vi "Dashboard Main.vi"() -> ()   [LabVIEW 2019]
uses:
  <vilib>/Utility/miscctls.llb/LVRowAndColumnTypeDef.ctl
  <vilib>/event_ctls.llb/eventvkey.ctl
  <vilib>/Rock Robotics/Network Tables/NT Read Numeric Array.vi
  <vilib>/Rock Robotics/Network Tables/NT Read Boolean.vi
  <vilib>/Rock Robotics/WPI/Dashboard/WPI_DashboardLogging Global.vi
panel:
  in  "Camera Settings Right":T1={"Frame Rate"=30, "Compression"=30, "Size"=1, "DB Camera Config"=FALSE} {"Frame Rate" scale=1.0..30.0; "Compression" scale=100.0..-1.0; "Size" items=["640x480", "320x240", "160x120"]}
  in  "Camera Name Right":string(combo)="No Camera Selection"
  out "Camera Perf":string
  in  "Camera Settings":T1={"Frame Rate"=30, "Compression"=30, "Size"=1, "DB Camera Config"=FALSE} {"Frame Rate" scale=1.0..30.0; "Compression" scale=100.0..-1.0; "Size" items=["640x480", "320x240", "160x120"]}
  in  "TCP":refnum<k5>
  in  "Rec Mode":enum32{"Stop", "Record", "Playback"}(radio)
  out "Robot IP":string
  out "Image Message":string="Timeout in Camera Communications"
  in  "Dashboard Tab":T2(tab)
  in  "Select Auto":string(combo)="Select Autonomous ..."
  out "NT Connection":bool
  out "MotorChart R":cluster{"Numeric":dbl, "Numeric":dbl}(graph)
  out "MotorChart L":cluster{"Numeric":dbl, "Numeric":dbl}(graph)
  out "MotorSliders R":cluster{"MotorSlide1":dbl, "MotorSlide2":dbl} {"MotorSlide2" scale=-1.0..1.0 scale format="%#_2e"; "MotorSlide1" scale=-1.0..1.0 scale format="%#_2e"}
  out "MotorSliders L":cluster{"MotorSlide1":dbl, "MotorSlide2":dbl} {"MotorSlide2" scale=-1.0..1.0 scale format="%#_2e"; "MotorSlide1" scale=-1.0..1.0 scale format="%#_2e"}
  out "Gyro":dbl(knob) scale=0.0..360.0
  out "JS1 Z":dbl(slide) scale=-1.0..1.0 scale format="%#_2e"
  out "JS1 Graph":cluster{"X":dbl, "Y":dbl}[](graph)
  out "JS1 Buttons":T3
  out "JS2 Z":dbl(slide) scale=-1.0..1.0 scale format="%#_2e"
  out "JS2 Graph":cluster{"X":dbl, "Y":dbl}[](graph)
  out "JS2 Buttons":T3
  out "Mode":T4(ring)=enum."Auto Disabled"
  out "Right Camera Perf":cluster{"Bandwidth (Mbps)":dbl, "FPS":dbl}
  out "Camera Image Right":T5(plugin-control)
  in  "DB/String 9":string
  in  "DB/String 8":string
  in  "DB/String 7":string
  in  "DB/String 6":string
  in  "DB/String 5":string
  in  "DB/String 4":string
  in  "DB/String 3":string
  in  "DB/String 2":string
  in  "DB/String 1":string
  in  "DB/String 0":string
  in  "DB/Slider 0":dbl(slide) scale=0.0..5.0
  in  "DB/Slider 1":dbl(slide) scale=0.0..5.0
  in  "DB/Slider 2":dbl(slide) scale=0.0..5.0
  in  "DB/Slider 3":dbl(slide) scale=0.0..5.0
  out "DB/LED 3":bool
  out "DB/LED 2":bool
  out "DB/LED 1":bool
  out "DB/LED 0":bool
  in  "DB/Button 3":bool
  in  "DB/Button 2":bool
  in  "DB/Button 1":bool
  in  "DB/Button 0":bool caption="New Name"
  out "Intake rotation":dbl(knob) scale=-100.0..100.0
  out "version_note":string
  in  "FIRE PULSE":dbl=0.4 caption="PULSE (s)" min=0.1 max=1.0 step=0.05 format="%#.1g"
  in  "FIRE SPD":dbl=0.4 min=0.4 max=1.0 step=0.1 format="%#.1g"
  out "GAME COLOR":u32(colorbox)
  out "SENSOR COLOR":u32(colorbox)
  out "DRIVER Z":dbl
  out "DRIVER Y":dbl
  out "SHOOTER HT":dbl[](array[slide]) caption="SHOOTER Ht & Spd" scale=0.2..1.0
  out "CW ROTATION":bool
  out "CW DEPLOY":bool
  out "LIFT LOCK":bool
  out "INV DRIVE":bool
  out "FORZA":bool
  out "1 Joystick":bool
  out "NEO MOTOR TEMPS":dbl[](array[slide]) scale=70.0..300.0
  in  "HEIGHT":i32
  in  "TOP":i32
  in  "WIDE":i32
  in  "LEFT":i32
  in  "Test Slider":dbl(slide) scale=0.0..100.0 scale format="%#_3g"
  in  "On/Off":bool caption="Solenoid"
  in  "Test Name":u16(ring) items=["Select the test to run..."]
  in  "Test Tree":string(tree)
  in  "Motor":cluster{"Value":dbl, "Enable":bool} {"Value" scale=-1.0..1.0 scale format="%#_3g"}
  out "Progress":T6 {"Test Progress" scale=0.0..100.0}
  in  "Rev/Fwd":cluster{"Forward":bool, "Reverse":bool}
  in  "Test Ring":u16(ring) items=["Monochrome", "Color"]
  out "Cmd Status":string
  in  "Execute Command":bool
  in  "Command Params":string[][](table)
  in  "Command Selection":i32(listbox)
  in  "CheckList":i32(listbox)
  out "Tree":string(tree)
  out "Camera Image":T5(plugin-control)
  out "Background":bool
  in  "Camera Name":string(combo)="No Camera Selection"
  # "HW"
  # "HW"
  # "Joysticks"
  # "Drive Motors"
  # "Front"
  # "Right"
  # "Left"
  # "Back"
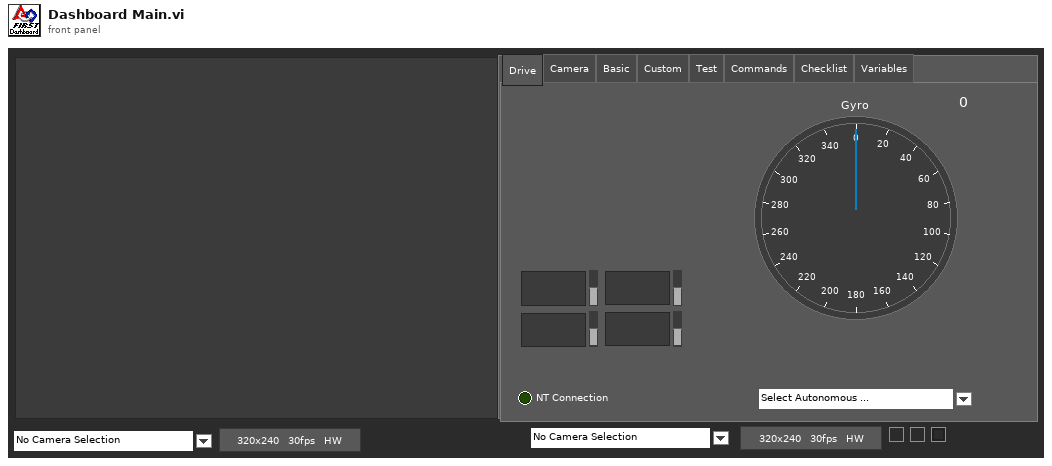
[diagram p1: front panel]
types:
  T1 = cluster{"Frame Rate":i32, "Compression":i32, "Size":u16, "DB Camera Config":bool}
  T2 = enum32{"Drive", "Camera", "Basic", "Custom", "Test", "Commands", "Checklist", "Variables"}
  T3 = cluster{bool, bool, bool, bool, bool, bool, bool, bool, bool, bool, bool, bool}
  T4 = enum8{"Tele-Op Disabled", "Tele-Op Enabled", "Auto Disabled", "Auto Enabled", "Test Disabled", "Test Enabled", "Disconnected", "No Code", "E-Stop"}
  T5 = typedef "IMAQ Image.ctl" = refnum<image>
  T6 = cluster{"Test Progress":u8, "Test Progress Text":string}
  T7 = cluster{"Save Path":path, "Interval (s)":dbl, "Keep":i32}
  T8 = typedef "Image Type" = u32
  T9 = cluster{"IDs":cluster{"RPC field ID":u16, "Unique ID":u16}, "String":string}
  T10 = cluster{"Error Strings":string, "Disable Counts":cluster{u16, u16}, "Rail Faults":cluster{u16, u16, u16}, "Robot IP":string, "DB Mode":u8, "Event Info":cluster{"Name":string, "Type":u8, "Number":u16, "Replay":u8}}
  T11 = cluster{"Storage":cluster{"Disk Free":u64, "RAM Block":u32, "RAM free":u32}, "CPU Utilization":cluster{"CPU % ISR":sgl, "CPU % Time Crit":sgl, "CPU % Timed Str":sgl, "CPU % High":sgl, "CPU % Above":sgl, "CPU % Normal":sgl, "CPU % Low":sgl}, "CAN":cluster{"% Bus Utilization":sgl, "Bus Off Cnt":u32, "TX_FIFO Full Cnt":u32, "Receive Error Cnt":u8, "Transmit Error Cnt":u8}, "HID":cluster{"HID Outputs":u32, "Rumble Low":u16, "Rumble High":u16}[]}
  T12 = cluster{"Status bits":cluster{"Test Mode":bool, "Autonomous":bool, "Enabled":bool, "Code Start":bool, "Brownout":bool, "Reserved 2":bool, "Reserved 3":bool, "E-Stop":bool}, "Code Trace":cluster{"Disabled":bool, "TeleOp":bool, "Auto":bool, "Test":bool}, "Controller Type":enum16{"unknown", "cRIO", "roboRio"}, "Code?":enum16{"unknown", "noCode", "code"}, "Battery V":dbl}
  T13 = cluster{"Control Bits":cluster{"TestMode":bool, "Autonomous":bool, "Enabled":bool, "FMS Present":bool, bool, bool, bool, "E-Stop":bool}, "Team Station ":u8, "Countdown":sgl, "Joystick Values":cluster{"Axes":dbl[], "Buttons":bool[], "POVs":i16[]}[]}
  T14 = cluster{"Axes":dbl[], "Buttons":bool[], "POVs":i16[]}[]
  T15 = cluster{"Axes":dbl[], "Buttons":bool[], "POVs":i16[]}
  T16 = cluster{"Buttons[0]":bool, "Buttons[1]":bool, "Buttons[2]":bool, "Buttons[3]":bool, "Buttons[4]":bool, "Buttons[5]":bool, "Buttons[6]":bool, "Buttons[7]":bool, "Buttons[8]":bool, "Buttons[9]":bool, "Buttons[10]":bool, "Buttons[11]":bool}
  T17 = cluster{"Camera Image":refnum<vi>, "Dashboard Tab":refnum<vi>, "Background":refnum<vi>, "Rec Mode":refnum<vi>, "Test Slider":refnum<vi>, "On/Off ":refnum<vi>, "Test Ring":refnum<vi>, "Rev/Fwd":refnum<vi>, "Test Name":refnum<vi>, "Motor":refnum<vi>, "Progress":refnum<vi>, "CheckList":refnum<vi>, "Tree":refnum<vi>, "Test Tree":refnum<vi>, "Command Params":refnum<vi>, "Command Selection":refnum<vi>, "Execute Command":refnum<vi>, "Cmd Status":refnum<vi>, "Camera Settings":refnum<vi>, "Camera Name":refnum<vi>, "Camera Perf":refnum<vi>, "Camera Settings Right":refnum<vi>, "Camera Name Right":refnum<vi>, "Camera Image Right":refnum<vi>}
  T18 = cluster{"Global Rectangle":i32[], "Contours":cluster{"Contour Type":u32, "ROI Type":u32, "Points":i32[]}[]}
  T19 = cluster{"Left":i32, "Top":i32, "Right":i32, "Bottom":i32}
  T20 = cluster{"Camera Name":string, string, "Saved DB Images Info":cluster{"Save Path":path, "Interval (s)":dbl, "Keep":i32}}
  T21 = cluster{"Camera Name Right":string, string, "Saved DB Images Info":cluster{"Save Path":path, "Interval (s)":dbl, "Keep":i32}}
  T22 = cluster{"Operation":enum16{"Update", "Clear"}, "Color Box":u32}[]
  T23 = typedef "eventvkey.ctl" = enum16{"ASCII", "Enter", "Return", "Shift", "Ctrl", "Alt", "Cmd", "Opt", "Caps", "NumLock", "Clear", "Break", "Up", "Down", "Left", "Right", "Insert", "Delete", "Home", "End", "PageUp", "PageDown", "Escape", "Help", "Pause", "ScrollLock", "F1", "F2", "F3", "F4", "F5", "F6", "F7", "F8", "F9", "F10", "F11", "F12", "F13", "F14", "F15", "F16", "F17", "F18", "F19", "F20", "F21", "F22", "F23", "F24", "Play", "VolumeUp", "VolumeDown", "Mute", "Two Byte Char"}
  T24 = cluster{"Image Size":bool, "Image Type":bool, "Pixel Value":bool, "ROI Information":bool, "Zoom Factor":bool}
  T25 = cluster{"Operation":enum16{"Update", "Clear"}, "Color Box":u32}
  T26 = typedef "LVRowAndColumnTypeDef.ctl" = cluster{"Row":i32, "Column":i32}
  T27 = cluster{"Shift":bool, "Ctrl":bool, "Alt":bool, "Cmd":bool, "Opt":bool}
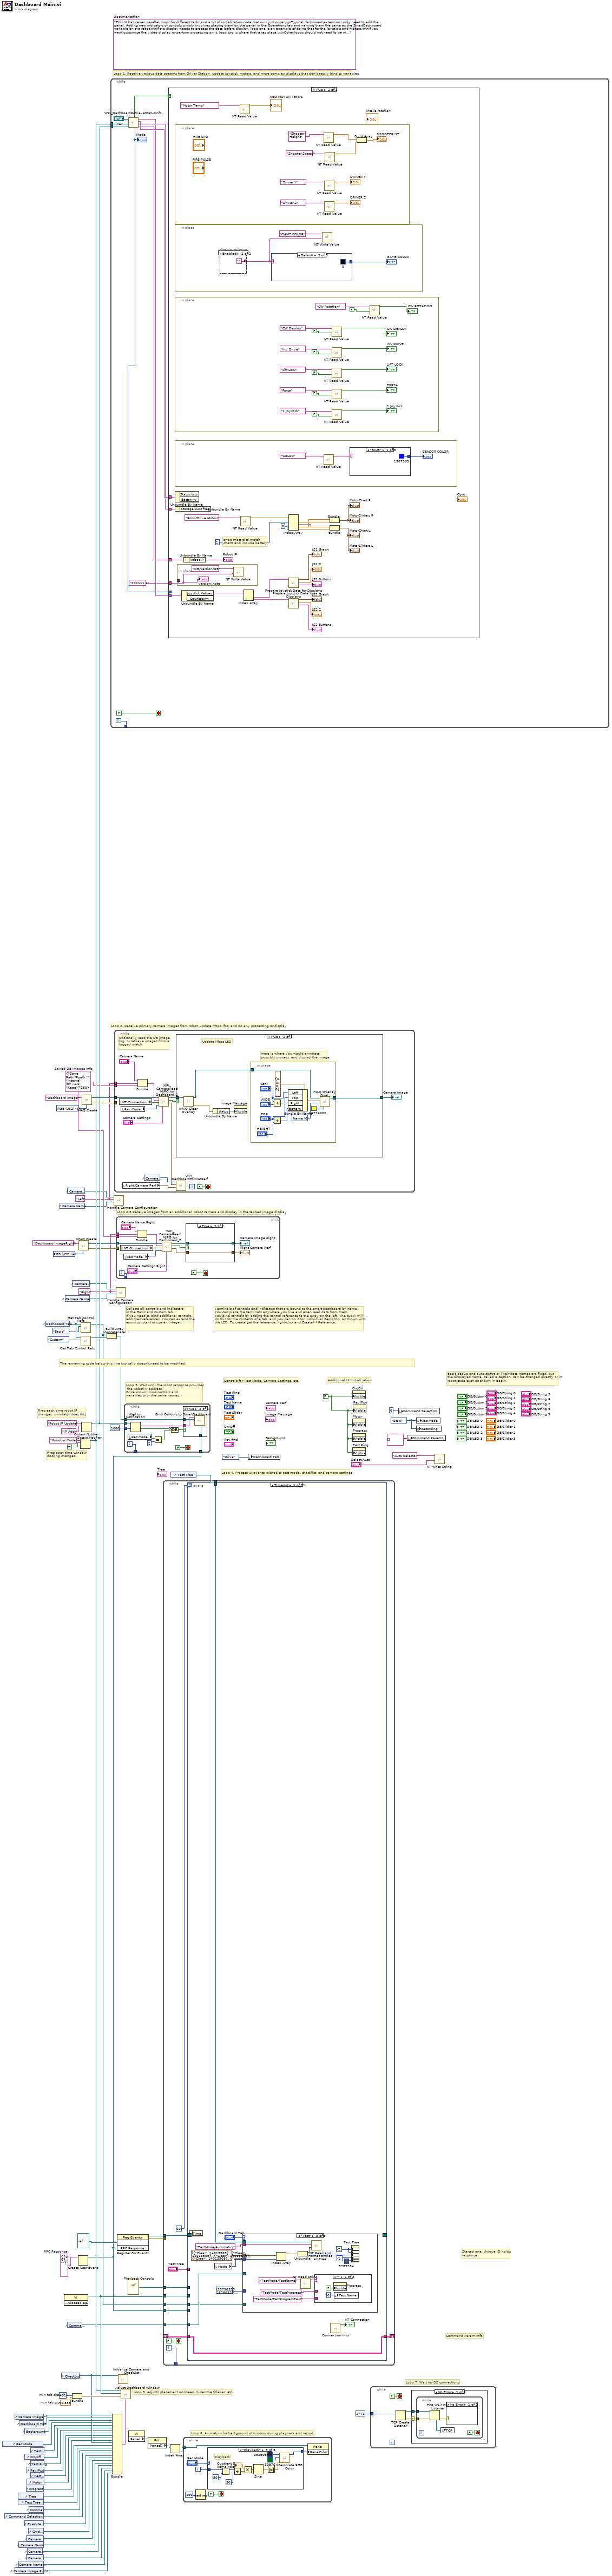
[diagram p0: block diagram]
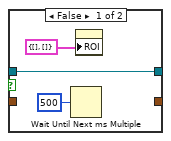
[diagram p2: hidden frame]
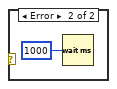
[diagram p3: hidden frame]
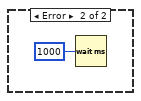
[diagram p4: hidden frame]
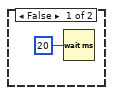
[diagram p5: hidden frame]
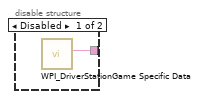
[diagram p6: hidden frame]
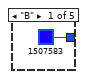
[diagram p7: hidden frame]
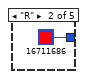
[diagram p8: hidden frame]
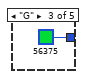
[diagram p9: hidden frame]
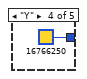
[diagram p10: hidden frame]
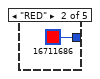
[diagram p11: hidden frame]
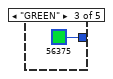
[diagram p12: hidden frame]
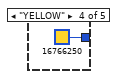
[diagram p13: hidden frame]
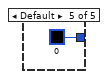
[diagram p14: hidden frame]
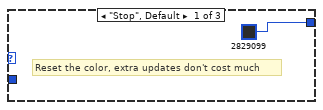
[diagram p15: hidden frame]
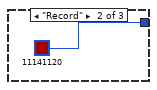
[diagram p16: hidden frame]
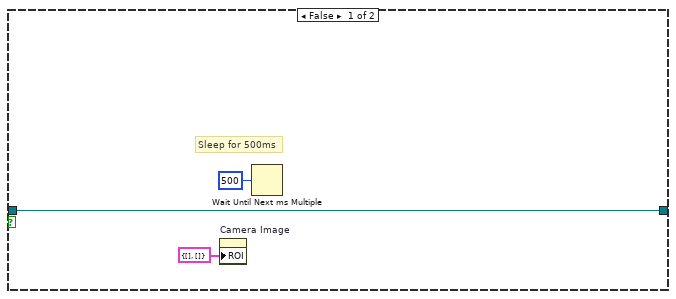
[diagram p18: hidden frame]
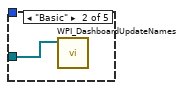
[diagram p20: hidden frame]
diagram:
  w3 = T7 {"Save Path"=path "", "Interval (s)"=1.0, "Keep"=180}  # Saved DB Images Info
  w2 = "Right"
  w1 = "Left"
  w13 = T8 4 items=["Grayscale (U8)", "Grayscale (I16)", "Grayscale (SGL)", "Complex (CSG)", "RGB (U32)", "HSL (U32)", "RGB (U64)"] ("Image Type")
  w29 = T9 {"IDs"={"RPC field ID"=0, "Unique ID"=0}, "String"=""}  # RPC Response
  w52 = 491  # min tab size
  w51 = 1.333  # min tab size
  w59 = enum32{"Stop", "Record", "Playback"}."Stop" ("Rec Mode")
  w36 = FALSE ("Visible")
  (unwired) "This VI has seven parallel loops for different tasks and a bit of initialization code that runs just once.\n\nTypical dashboard extensions only need to edit the panel. Adding new indicators or controls simply involves placing them on the panel in the Operations tab and naming them the same as the SmartDashboard variable on the robot\n\nIf the display needs to process the data before display, loop one is an example of doing that for the joysticks and motors.\n\nIf you want customize the video display or perform processing on it, loop two is where that takes place.\n\nOther loops should not need to be modified. They are pretty standard, and document the task they perform."  # Documentation
  w76 = T8 4 items=["Grayscale (U8)", "Grayscale (I16)", "Grayscale (SGL)", "Complex (CSG)", "RGB (U32)", "HSL (U32)", "RGB (U64)"] ("Image Type")
  # "Loop 2.5 Receive images from an additional  robot camera and display in the tabbed image display"
  # "Command Param Info"
  # "Started one, Unique ID holds\nresponse"
  # "Loop 7. Wait for DS connections"
  # "Basic debug and auto controls: Their data names are fixed, but\nthe displayed name, called a caption, can be changed directly or in\nrobot code such as shown in Begin."
  # "Controls for Test Mode, Camera Settings, etc."
  # "Additional UI Initialization"
  # "Loop 6. Animation for background of window during playback and record"
  # "Fires each time robot IP\nchanges, simulator does this"
  # "Fires each time window\ndocking changes."
  # "Collects all controls and indicators\nin the Basic and Custom tab.\nIf you need to bind additional controls,\nadd their references. You can extend the\nenum constant or use an integer."
  # "The remaining code below this line typically doesn't need to be modified."
  # "Loop 4. Process UI events related to test mode, checklist, and camera settings"
  # "Terminals of controls and indicators that are bound to the smart dashboard by name.\nYou can place the terminals anywhere you like and even read data from them.\nYou bind controls by adding the control reference to the array on the left. The subVI will\ndo this for the contents of a tab, and you can do it for individual items too, as shown with\nthe LED. To create get the reference, right-click and Create>>Reference."
  # "Loop 3. Wait until the robot response provides\n the Robot IP address.\nOnce known, bind controls and\nvariables with the same names."
  # "Loop 5. Adjusts placement onscreen, hides the titlebar, etc."
  # "Loop 1. Receive various data streams from Driver Station, update joystick, motors, and more complex displays that don't easily bind to variables."
  # "Loop 2. Receive primary camera images from robot, update Mbps, fps, and do any processing or display"
  n1 = control-ref of="Rec Mode"() -> (w42:refnum<vi>)
  n2 = control-ref of="Command Selection"() -> (w28:refnum<vi>)
  n3 = control-ref of="Camera Image Right"() -> (w6:refnum<vi>)
  n4 = control-ref of="Camera Image"() -> (w54:refnum<vi>)
  n5 = control-ref of="Tree"() -> (w46:refnum<vi>)
  n6 = control-ref of="Test Tree"() -> (w45:refnum<vi>)
  n7 = control-ref of="Camera Name"() -> (w19:refnum<vi>)
  n8 = control-ref of="Camera Name Right"() -> (w7:refnum<vi>)
  n9 = control-ref of="Dashboard Tab"() -> (w53:refnum<vi>)
  n10 = control-ref of="Execute Command"() -> (w30:refnum<vi>)
  n11 = control-ref of="Background"() -> (w49:refnum<vi>)
  n12 = control-ref of="On/Off"() -> (w40:refnum<vi>)
  n13 = control-ref of="Progress"() -> (w37:refnum<vi>)
  n14 = control-ref of="Camera Settings"() -> (w20:refnum<vi>)
  n15 = control-ref of="Camera Settings Right"() -> (w8:refnum<vi>)
  n16 = control-ref of="Rev/Fwd"() -> (w38:refnum<vi>)
  n17 = control-ref of="Motor"() -> (w43:refnum<vi>)
  n18 = control-ref of="Camera Perf"() -> (w18:refnum<vi>)
  n19 = control-ref of="Cmd Status"() -> (w24:refnum<vi>)
  n20 = control-ref of="Command Params"() -> (w31:refnum<vi>)
  n21 = control-ref of="Test Slider"() -> (w41:refnum<vi>)
  n22 = control-ref of="Test Ring"() -> (w39:refnum<vi>)
  n23 = control-ref of="Test Name"() -> (w44:refnum<vi>)
  n24 = control-ref of="Dashboard Tab"() -> (w57:refnum<vi>)
  n25 = control-ref of="Camera Name"() -> (w21:refnum<vi>)
  n26 = control-ref of="CheckList"() -> (w47:refnum<vi>)
  n27 = property class="VI" props=["Front Panel.Closeable"]() -> (reference out=w58:refnum<vi>)  [unwired: 2 in, 2 out]
  n28 = control-ref of="Camera Name Right"() -> (w9:refnum<vi>)
  n29 = control-ref of="Camera Settings"() -> (w22:refnum<vi>)
  n30 = control-ref of="Command Params"() -> (w23:refnum<vi>)
  n31 = control-ref of="Camera Settings Right"() -> (w10:refnum<vi>)
  n32 = Bundle("min tab size"=w52, "min tab size"=w51) -> (w50:cluster{"min tab size":i32, "min tab size":dbl})  [unwired: 1 in]
  n33 = Create User Event(user event datatype=w29) -> (user event=w25:refnum<user-event>)  [unwired: 1 in, 1 out]
  n34 = call "IMAQ Create"("Image Name"="Dashboard ImageRight", "Image Type"=w13) -> ("New Image"=w12:T5, "error out"=w11:errorcluster)  [unwired: 2 in, 1 out]
  n35 = Obtain Notifier(name (unnamed)="Window Mode", notification data type=TRUE) -> (notifier out=w34:refnum<notifier>)  [unwired: 2 in, 2 out]
  n36 = call <vilib>:"Get Tab Control Refs.vi"("Page Index"=T2."Basic" ("Dashboard Tab"), "TabControl in"=w57) -> ("ControlsOnPage"=w17:refnum<vi>[])  [unwired: 9 in]
  n37 = call <vilib>:"Get Tab Control Refs.vi"("Page Index"=T2."Custom" ("Dashboard Tab"), "TabControl in"=w57) -> ("ControlsOnPage"=w56:refnum<vi>[])  [unwired: 9 in]
  n38 = Obtain Notifier(name (unnamed)="Robot IP Update", notification data type="IP Addr" ("name (unnamed)")) -> (notifier out=w35:refnum<notifier>)  [unwired: 2 in, 2 out]
  n39 = call "IMAQ Create"("Image Name"="Dashboard Image", "Image Type"=w76) -> ("New Image"=w74:T5, "error out"=w73:errorcluster)  [unwired: 2 in, 1 out]
  n40 = Build Array (concatenate)(w17, w56) -> (w55:refnum<vi>[])
  n41 = while {
    tunnel: [w87] -> _
    tunnel: w35 -> [w81]
    tunnel: w34 -> [w78]
    i -> [w87]
    stop <- FALSE stop-if-true
    n42 = call <vilib>:"WPI_DashboardRetrieveStatusInfo.vi"("Binding Refnum"=w81, "Window Mode Notifier"=w78, "TCP Cnx"="TCP") -> ("Power and Errors"=w82:T10, "Robot Metrics"=w85:T11, "Status Info"=w86:T12, "Control Info"=w83:T13, "Robot Mode"=w80:T4, "Process?"=w84:bool)  [unwired: 3 in]
    "Mode" <- w80
    n43 = case shown="True" w84 {
      tunnel: w86 -> [_ w116]
      tunnel: w85 -> [_ w115]
      tunnel: w83 -> [_ w114]
      tunnel: w82 -> [_ w113]
      tunnel: w80 -> [_ _]
      tunnel: "2021v1.2" ("version_note") -> [_ w92]
      frame False {
        n44 = Wait (ms)(milliseconds to wait=u32 20) -> ()  [unwired: 1 out]
      }
      frame True {
        # "swap motors to match\ncharts and include battery"
        n45 = in-place {
          n46 = call-poly <vilib>:"NT Read Value.vi"("Name"="Shooter Height") -> ("Numeric"=w140:dbl)  [unwired: 9 in, 1 out]
          n47 = call-poly <vilib>:"NT Read Value.vi"("Name"="Driver Y") -> ("Numeric"=→"DRIVER Y":dbl)  [unwired: 9 in, 1 out]
          n48 = call-poly <vilib>:"NT Read Value.vi"("Name"="Driver Z") -> ("Numeric"=→"DRIVER Z":dbl)  [unwired: 9 in, 1 out]
          n49 = call-poly <vilib>:"NT Read Value.vi"("Name"="Shooter Speed") -> ("Numeric"=w138:dbl)  [unwired: 9 in, 1 out]
          n50 = Build Array(w140, w138) -> (→"SHOOTER HT":dbl[])
        }
        n51 = in-place {
          n52 = disable-structure shown="Enabled" {
            disable-tunnel: [w122 "" ("Game Specific Data")] -> w119
            frame Disabled {
              n53 = call <vilib>:"WPI_DriverStationGame Specific Data.vi"() -> ("Game Specific Data"=w122:string)  [unwired: 11 in]
            }
            frame Enabled {
            }
          }
          n54 = case shown="Default" w119 {
            tunnel: [u32 1507583 ("SENSOR COLOR") u32 16711686 ("SENSOR COLOR") u32 56375 ("SENSOR COLOR") u32 16766250 ("SENSOR COLOR") u32 0 ("SENSOR COLOR")] -> w121
            frame "B" {
            }
            frame "R" {
            }
            frame "G" {
            }
            frame "Y" {
            }
            frame Default {
            }
          }
          "GAME COLOR" <- w121
          n55 = call-poly <vilib>:"NT Write Value.vi"("String"=w119, "Name"="GAME COLOR") -> ()  [unwired: 9 in, 1 out]
        }
        n56 = in-place {
          n57 = call-poly <vilib>:"NT Read Value.vi"("Default Value"=FALSE, "Name"="CW Deploy") -> ("Boolean"=→"CW DEPLOY":bool)  [unwired: 8 in, 1 out]
          n58 = call-poly <vilib>:"NT Read Value.vi"("Default Value"=FALSE, "Name"="Inv Drive") -> ("Boolean"=→"INV DRIVE":bool)  [unwired: 8 in, 1 out]
          n59 = call-poly <vilib>:"NT Read Value.vi"("Default Value"=FALSE, "Name"="Lift Lock") -> ("Boolean"=→"LIFT LOCK":bool)  [unwired: 8 in, 1 out]
          n60 = call-poly <vilib>:"NT Read Value.vi"("Default Value"=FALSE, "Name"="Forza") -> ("Boolean"=→"FORZA":bool)  [unwired: 8 in, 1 out]
          n61 = call-poly <vilib>:"NT Read Value.vi"("Default Value"=FALSE, "Name"="1 Joystick") -> ("Boolean"=→"1 Joystick":bool)  [unwired: 8 in, 1 out]
          n62 = call-poly <vilib>:"NT Read Value.vi"("Default Value"=FALSE, "Name"="CW Rotation") -> ("Boolean"=→"CW ROTATION":bool)  [unwired: 8 in, 1 out]
        }
        n63 = in-place {
          n64 = call-poly <vilib>:"NT Read Value.vi"("Name"="COLOR") -> ("String"=w130:string)  [unwired: 9 in, 1 out]
          n65 = case shown="\"BLUE\"" w130 {
            tunnel: [u32 1507583 ("SENSOR COLOR") u32 16711686 ("SENSOR COLOR") u32 56375 ("SENSOR COLOR") u32 16766250 ("SENSOR COLOR") u32 0 ("SENSOR COLOR")] -> w129
            frame "BLUE" {
            }
            frame "RED" {
            }
            frame "GREEN" {
            }
            frame "YELLOW" {
            }
            frame Default {
            }
          }
          "SENSOR COLOR" <- w129
        }
        n66 = Unbundle By Name(w116) -> ()  [unwired: 2 out]
        n67 = Unbundle By Name(w115) -> ()  [unwired: 1 out]
        n68 = in-place {
          in-place-border: w92 -> [w117]
          n69 = call-poly <vilib>:"NT Write Value.vi"("String"=w117, "Name"="DB/version/DB") -> ()  [unwired: 9 in, 1 out]
          "version_note" <- w117
        }
        n70 = Unbundle By Name(w114) -> ("Joystick Values"=w104:T14)  [unwired: 1 out]
        n71 = Unbundle By Name(w113) -> ("Robot IP"=→"Robot IP":string)
        n72 = call-poly <vilib>:"NT Read Value.vi"("Name"="Motor Temp") -> ("Numeric Array"=→"NEO MOTOR TEMPS":dbl[])  [unwired: 9 in, 1 out]
        n73 = call-poly <vilib>:"NT Read Value.vi"("Name"="RobotDrive Motors") -> ("Numeric Array"=w94:dbl[])  [unwired: 9 in, 1 out]
        n74 = Index Array(array=w104) -> (element #1=w103:T15, element #2=w99:T15)  [unwired: 2 in]
        n75 = Index Array(array=w94, index #1=1, index #4=0) -> (element #1=w108:dbl, element #2=w109:dbl, element #3=w107:dbl, element #4=w112:dbl)  [unwired: 2 in]
        n76 = call "Prepare Joystick Data for Displays.vi"("Joystick Values"=w103) -> ("Buttons"=→"JS1 Buttons":T16, "Z Axis"=→"JS1 Z":dbl, "Cartesian Data"=→"JS1 Graph":cluster{"X axis":dbl, "X axis":dbl}[])  [unwired: 8 in]
        n77 = call "Prepare Joystick Data for Displays.vi"("Joystick Values"=w99) -> ("Buttons"=→"JS2 Buttons":T16, "Z Axis"=→"JS2 Z":dbl, "Cartesian Data"=→"JS2 Graph":cluster{"X axis":dbl, "X axis":dbl}[])  [unwired: 8 in]
        n78 = Bundle("Numeric"=w107, "Numeric"=w108) -> (→"MotorChart R" →"MotorSliders R":cluster{"Numeric":dbl, "Numeric":dbl})  [unwired: 1 in]
        n79 = Bundle("Numeric"=w109, "Numeric"=w112) -> (→"MotorChart L" →"MotorSliders L":cluster{"Numeric":dbl, "Numeric":dbl})  [unwired: 1 in]
      }
    }
  }
  n80 = Bundle("Camera Image"=w54, "Dashboard Tab"=w53, "Background"=w49, "Rec Mode"=w42, "Test Slider"=w41, "On/Off"=w40, "Test Ring"=w39, "Rev/Fwd"=w38, "Test Name"=w44, "Motor"=w43, "Progress"=w37, "CheckList"=w47, "Tree"=w46, "Test Tree"=w45, "Command Params"=w31, "Command Selection"=w28, "Execute Command"=w30, "Cmd Status"=w24, "Camera Settings"=w20, "Camera Name"=w19, "Camera Perf"=w18, "Camera Settings Right"=w8, "Camera Name Right"=w7, "Camera Image Right"=w6) -> (w48:T17)  [unwired: 1 in]
  n81 = call "Handle Camera Configuration.vi"("CameraNameRef"=w21, "Display Name"=w1, "ClusterRef"=w22) -> ()  [unwired: 9 in]
  n82 = while {
    tunnel: w74 -> [w177]
    tunnel: w73 -> [_]
    tunnel: w3 -> [w170]
    tunnel: w1 -> [w167]
    stop <- FALSE stop-if-true
    # "Optionally read the DB image,\nlog, or retrieve images from a\nlogged match"
    n83 = local read "NT Connection"() -> (w171:bool)
    n84 = local read "Rec Mode"() -> (w174:enum32{"Stop", "Record", "Playback"})
    n85 = local read "Right Camera Perf"() -> (w165:cluster{"Bandwidth (Mbps)":dbl, "FPS":dbl})
    n86 = Bundle("Camera Name"="Camera Name", w167, "Saved DB Images Info"=w170) -> (w169:T20)  [unwired: 1 in]
    n87 = control-ref of="Camera Perf"() -> (w164:refnum<vi>)
    n88 = call <vilib>:"WPI_CameraRead MJPG for Dashboard_2.vi"("Camera Settings"="Camera Settings", "Rec Mode"=w174, "NT Connection"=w171, "Capture Info"=w169, "Image in"=w177) -> ("perf info"=w166:cluster{"Bandwidth (Mbps)":dbl, "fps":dbl}, "Active"=w175:bool, "Image\\ out"=w176:T5)  [unwired: 4 in]
    n89 = case shown="True" w175 {
      tunnel: w176 -> [w180 w184]
      tunnel: [w180 w182] -> w172
      frame False {
        # "Sleep for 500ms"
        n90 = property on="Camera Image" class="ImageControl"("ROI"=T18 {"Global Rectangle"=[], "Contours"=[]}) -> ()  [unwired: 2 in, 2 out]
        n91 = Wait Until Next ms Multiple(millisecond multiple=u32 500) -> ()  [unwired: 1 out]
      }
      frame True {
        # "Here is where you would annotate,\npossibly process, and display the image"
        # "Update Mbps LED"
        n92 = call "IMAQ Clear Overlay"("Image"=w184) -> ("error out"=w185:errorcluster, "Image Out"=w183:T5)  [unwired: 2 in, 7 out]
        n93 = Unbundle By Name(w185) -> ("status"=w186:bool)
        n94 = property on="Image Message" class="Str"("Visible"=w186) -> ()  [unwired: 2 in, 2 out]
        n95 = in-place {
          in-place-border: w183 -> [w198]
          in-place-border: [w197] -> w182
          w196 = u32 0 items=["Frame", "Fill"] ("Drawing Mode (Frame)")
          n96 = Add(x="LEFT", y="WIDE") -> (x+y=w193:i32)
          n97 = Add(x="TOP", y="HEIGHT") -> (x+y=w192:i32)
          n98 = Bundle By Name(cluster=T19 {"Left"=0, "Top"=0, "Right"=0, "Bottom"=0} ("Bounding Rectangle"), "Left"="LEFT", "Top"="TOP", "Right"=w193, "Bottom"=w192) -> (w194:T19)
          n99 = call "IMAQ Overlay Oval"("Color"=u32 16776002, "Drawing Mode (Frame)"=w196, "Bounding Rectangle"=w194, "Image"=w198) -> ("Image Out"=w197:T5)  [unwired: 6 in, 1 out]
        }
      }
    }
    "Camera Image" <- w172
    n100 = call <vilib>:"WPI_DashboardFormatPerf.vi"("Right Camera Perf"=w165, "Performance"=w166, "String in"=w164) -> ()  [unwired: 9 in]
  }
  n101 = call "Handle Camera Configuration.vi"("CameraNameRef"=w9, "Display Name"=w2, "ClusterRef"=w10) -> ()  [unwired: 9 in]
  n102 = while {
    tunnel: w12 -> [w213]
    tunnel: w11 -> [_]
    tunnel: [w208] -> _
    tunnel: w3 -> [w204]
    tunnel: w2 -> [w201]
    i -> [w208]
    stop <- FALSE stop-if-true
    n103 = local read "NT Connection"() -> (w205:bool)
    n104 = local read "Rec Mode"() -> (w212:enum32{"Stop", "Record", "Playback"})
    n105 = Bundle("Camera Name Right"="Camera Name Right", w201, "Saved DB Images Info"=w204) -> (w203:T21)  [unwired: 1 in]
    n106 = call <vilib>:"WPI_CameraRead MJPG for Dashboard_2.vi"("Camera Settings"="Camera Settings Right", "Rec Mode"=w212, "NT Connection"=w205, "Capture Info"=w203, "Image in"=w213) -> ("perf info"=w199:cluster{"Bandwidth (Mbps)":dbl, "fps":dbl}, "Active"=w207:bool, "Image\\ out"=w210:T5)  [unwired: 4 in]
    n107 = case shown="True" w207 {
      tunnel: w210 -> [w215 w218]
      tunnel: [w215 w218] -> w206
      tunnel: [_ w217] -> w200
      tunnel: w199 -> [_ w217]
      frame False {
        n108 = Wait Until Next ms Multiple(millisecond multiple=u32 500) -> ()  [unwired: 1 out]
        n109 = property on="Camera Image Right" class="ImageControl"("ROI"=T18 {"Global Rectangle"=[], "Contours"=[]}) -> ()  [unwired: 2 in, 2 out]
      }
      frame True {
      }
    }
    "Camera Image Right" <- w206
    "Right Camera Perf" <- w200
  }
  n110 = register-events(refnum<vi> refnum, w25) -> (reference out=w63:refnum<event-registration>, error out=w62:errorcluster)  [unwired: 2 in]
  n111 = call "Initialize Camera and CheckList.vi"("ListBox in"=w47) -> ()  [unwired: 11 in]
  n112 = call "Adjust Dashboard Window.vi"("Sizing Refnums"=w48, "Size Constraints"=w50, "VI"=w58, "WIn Mode"=w34) -> ()  [unwired: 8 in]
  n113 = while {
    tunnel: w55 -> [w230]
    tunnel: w35 -> [w228]
    tunnel: [w226] -> _
    tunnel: u32 1000 ("milliseconds to wait") -> [w225]
    tunnel: w25 -> [w219]
    i -> [w226]
    stop <- FALSE stop-if-true
    n114 = local read "Rec Mode"() -> (w221:enum32{"Stop", "Record", "Playback"})
    n115 = Wait on Notification(notifier=w228, timeout in ms (-1)=w225) -> (notification=w227:string, timed out?=w223:bool)  [unwired: 2 in, 2 out]
    n116 = Equal?(x=w221, y=u16 2 ("Rec Mode")) -> (x = y?=w222:bool)
    n117 = Compound Arithmetic op=OR(invert w223, w222) -> (w224:bool)
    n118 = case shown="True" w224 {
      tunnel: w230 -> [_ w233]
      tunnel: w227 -> [_ w232]
      tunnel: w219 -> [_ w231]
      frame False {
      }
      frame True {
        n119 = call <vilib>:"Bind Controls to SmartDashboard.vi"("RPC ref"=w231, "Bound Control Refs"=w233, "Server IP Address"=w232) -> ()  [unwired: 9 in]
      }
    }
  }
  n120 = vi-ref "Playback Controls.vi"() -> (w64:refnum<vi>)
  n121 = property class="VI"() -> ("Panel"=w66:refnum<vi>)  [unwired: 2 in, 2 out]
  n122 = property class="Pnl"(reference=w66) -> ("Panes[]"=w67:refnum<vi>[])  [unwired: 1 in, 2 out]
  n123 = Index Array(array=w67) -> (element=w65:refnum<vi>)  [unwired: 1 in]
  n124 = control-ref of="Test Tree"() -> (w68:refnum<vi>)
  n125 = while {
    tunnel: [w243] -> _
    tunnel: w68 -> [w242]
    tunnel: w64 -> [w241]
    tunnel: w63 -> [w240]
    tunnel: w62 -> [_]
    tunnel: w58 -> [w239]
    tunnel: w25 -> [w238]
    tunnel: w23 -> [w237]
    shift-right: [w236] -> _
    shift-left: _ -> [w235]
    tunnel: w17 -> [w234]
    i -> [w243]
    stop <- FALSE stop-if-true
    n126 = event shown="[0] Timeout" {
      selector: w240 -> [_ _ _ _ _ _ _ _ _ _ _ _ _ _ _ _ _ _ _ _ _]
      dyn-events: [_ _ _ _ _ _ _ _ _ _ _ _ _ _ _ _ w503 _ _ _ _] -> _
      timeout: u32 60 ("milliseconds to wait") -> [_ _ _ _ _ _ _ _ _ _ _ _ _ _ _ _ _ _ _ _ _]
      tunnel: w242 -> [w255 _ _ _ _ _ _ _ _ _ _ _ _ _ _ _ _ _ _ _ _]
      tunnel: "Test Tree" -> [_ _ _ _ _ _ _ _ _ _ _ w470 w478 w480 w484 w492 _ _ _ _ _]
      tunnel: w241 -> [_ _ _ _ _ _ _ _ _ _ _ _ _ _ _ _ w505 _ w523 _ _]
      tunnel: w239 -> [_ _ _ _ _ _ _ _ _ _ _ _ _ _ _ _ w501 _ _ _ _]
      tunnel: w238 -> [_ _ _ _ _ _ _ _ _ _ _ _ _ _ _ _ w499 _ _ _ _]
      tunnel: w237 -> [w250 _ _ _ _ _ w421 _ _ _ _ _ _ _ _ _ _ _ _ _ _]
      tunnel: [w249 w298 w400 w405 w414 w418 w419 w428 w438 w445 w457 w469 w476 w479 w483 w491 w498 w518 w520 w524 w537] -> w236
      tunnel: w235 -> [w249 w298 w400 w405 w414 w418 w419 _ _ w445 w457 w469 w476 w479 w483 w491 w498 w518 w520 w524 w537]
      tunnel: w234 -> [w247 _ _ _ _ _ _ _ _ _ _ _ _ _ _ _ _ _ _ _ _]
      event Timeout {
        n127 = event-data() -> ()  [unwired: 1 in, 1 out]
        n128 = local read "Mode"() -> (w252:T4)
        n129 = case shown="\"Test\"" "Dashboard Tab" {
          tunnel: w255 -> [_ _ w271 _ _]
          tunnel: "TestMode/Automatic/" ("Name Pattern") -> [_ _ w270 _ _]
          tunnel: T22 [{"Operation"=enum."Clear", "Color Box"=14013909}, {"Operation"=enum."Clear", "Color Box"=14013909}, {"Operation"=enum."Clear", "Color Box"=14013909}, {"Operation"=enum."Clear", "Color Box"=14013909}, {"Operation"=enum."Update", "Color Box"=14013909}, {"Operation"=enum."Update", "Color Box"=16777215}, {"Operation"=enum."Clear", "Color Box"=14013909}, {"Operation"=enum."Clear", "Color Box"=14013909}, {"Operation"=enum."Clear", "Color Box"=14013909}] -> [_ _ w263 _ w291]
          tunnel: w252 -> [_ _ w262 _ w290]
          tunnel: u32[] [15790320, 15790320, 15790320, 15790320, 16777215, 16777215, 15790320, 15790320, 15790320] -> [_ _ _ _ w296]
          tunnel: w250 -> [_ _ _ _ w284]
          tunnel: w247 -> [_ w257 _ _ _]
          frame "Custom", Default {
          }
          frame "Basic" {
            n130 = call <vilib>:"WPI_DashboardUpdateNames.vi"("Controls on Tab"=w257) -> ()  [unwired: 11 in]
          }
          frame "Test" {
            w269 = -2 ("Active Item:Row Number")
            n131 = Index Array(array=w263, index=w262) -> (element=w264:T25)
            n132 = Unbundle(w264) -> ("Operation"=w265:enum16{"Update", "Clear"}, "Color Box"=w266:u32)
            n133 = call <vilib>:"NT Read String.vi"("Name"="TestMode/TestName") -> ("String"=w260:string)  [unwired: 9 in, 1 out]
            n134 = call <vilib>:"NT Read and Format Entries as Tree.vi"("Operation"=w265, "Name Pattern"=w270, "Tree Refnum"=w271) -> ()  [unwired: 7 in, 2 out]
            n135 = case shown="\"\"" w260 {
              tunnel: "TestMode/TestProgress" ("Name") -> [w273 _]
              tunnel: "TestMode/TestProgressText" ("Name") -> [w272 _]
              frame Default {
                n136 = call <vilib>:"NT Read Number.vi"("Name"=w273) -> ("Numeric"=w274:dbl)  [unwired: 9 in, 1 out]
                n137 = call <vilib>:"NT Read String.vi"("Name"=w272) -> ("String"=w275:string)  [unwired: 9 in, 1 out]
                n138 = Bundle("Numeric"=w274, "String"=w275) -> (→"Progress":cluster{"Numeric":dbl, "String":string})  [unwired: 1 in]
              }
              frame "" {
                n139 = property on="Progress" class="Clust (strict)"("Visible"=FALSE) -> ()  [unwired: 2 in, 2 out]
                n140 = local write "Test Name"(u16 0) -> ()
              }
            }
            n141 = property on="Test Tree" class="Tree (strict)"("Active Item Row Number"=w269, "ActiveColNum"=w269, "CellBG"=w266, "Active Item Row Number"=-1 ("Active Item:Row Number"), "CellBG"=u32 5789784 ("Color Box")) -> ()  [unwired: 2 in, 2 out]
          }
          frame "Variables" {
            w281 = string[] ["CameraPublisher", "Usage", "DB"]  # Items to initially close
            n142 = First Call?() -> (First Call?: T/F=w282:bool)
            n143 = control-ref of="Tree"() -> (w283:refnum<vi>)
            n144 = Select(t=w281, s=w282, f=string[] []) -> (s? t:f=w279:string[])
            n145 = call <vilib>:"NT Read and Format Entries as Tree.vi"("Tags to  Close"=w279, "Tree Refnum"=w283) -> ()  [unwired: 8 in, 2 out]
          }
          frame "Commands" {
            w292 = u32 5789784 ("Color Box")
            w293 = T26 {"Row"=-1, "Column"=-2} ("Active Cell:Active Cell")
            w295 = T26 {"Row"=-2, "Column"=-2} ("Active Cell:Active Cell")
            n146 = Index Array(array=w296, index=w290) -> (element=w294:u32)
            n147 = Index Array(array=w291, index=w290) -> (element=w289:T25)
            n148 = Unbundle(w289) -> ("Operation"=w288:enum16{"Update", "Clear"})  [unwired: 1 out]
            n149 = local read "Command Selection"() -> (w287:i32)
            n150 = property on="Command Selection" class="MCListbox (strict)"("ActiveCell"=w295, "CellBG"=w294, "ActiveCell"=w293, "CellBG"=w292) -> ()  [unwired: 2 in, 2 out]
            n151 = call <vilib>:"WPI_DashboardUpdate RPC Info.vi"("Operation"=w288) -> ("update"=w286:bool, "commands"=w285:string[][])  [unwired: 9 in]
            n152 = property on="Command Selection" class="MCListbox (strict)"("ItemNames"=w285) -> ()  [unwired: 2 in, 2 out]
            n153 = property on="Command Params" class="Tbl (strict)"("Active Cell"=w295, "Cell BG Color"=w294, "Active Cell"=w293, "Cell BG Color"=w292) -> ()  [unwired: 2 in, 2 out]
            n154 = call <vilib>:"WPI_DashboardUpdate Command Params.vi"("Update"=w286, "NewVal"=w287, "Commands"=w285, "Param Tbl"=w284) -> ()  [unwired: 7 in, 1 out]
          }
        }
        n155 = call <vilib>:"Connextion Info.vi"() -> ("Connected"=→"NT Connection":bool)  [unwired: 10 in, 1 out]
      }
      event "Test Tree": Value Change {
        # "Show appropriate\ncontrols"
        n156 = event-data() -> ("CtlRef"=w301:refnum<vi>, "NewVal"=w299:string)  [unwired: 1 in]
        n157 = call <vilib>:"WPI_UtilitiesGetTreeIOName.vi"("NewVal"=w299, "TreeControl in"=w301) -> ("I/O Name"=w302:string)  [unwired: 9 in]
        n158 = case shown="\"Camera\"" w302 {
          selector: w302 -> [_ w309 _ w331 w340 _]
          tunnel: w299 -> [_ _ w328 w330 _ w347]
          tunnel: cluster{string[]}[] [{["640x480", "320x240", "160x120"]}, {["Auto", "Fixed indoor", "Fixed outdoor 1", "Fixed outdoor 2", "Fixed fluorescent 1", "Fixed fluorescent 2", "Hold current"]}, {["Auto", "Flicker-free 50 Hz", "Flicker-free 60 Hz", "Hold current"]}, {["None", "Prioritize frame rate", "Prioritize image quality"]}, {["Monochrome", "Color"]}] -> [_ _ _ _ _ w346]
          frame Default {
            w304 = FALSE ("Visible")
            w303 = FALSE ("Visible")
            n159 = property on="Motor" class="Clust (strict)"("Visible"=w303) -> ()  [unwired: 2 in, 2 out]
            n160 = property on="Test Ring" class="Ring (strict)"("Visible"=w303) -> ()  [unwired: 2 in, 2 out]
            n161 = property on="Rev/Fwd" class="Clust (strict)"("Visible"=w304) -> ()  [unwired: 2 in, 2 out]
            n162 = property on="On/Off" class="Bool (strict)"("Visible"=w304) -> ()  [unwired: 2 in, 2 out]
            n163 = property on="Test Slider" class="Slide (strict)"("Visible"=w304) -> ()  [unwired: 2 in, 2 out]
          }
          frame "Analog Out", "Motor", "PWM" {
            w310 = FALSE ("Visible")
            n164 = case shown="\"Analog Out\"" w309 {
              tunnel: [1.0 ("Value") -1.0 ("Value") 0.0 ("Value")] -> w308
              tunnel: [255.0 ("Value") 1.0 ("Value") 5.0 ("Value")] -> w307
              tunnel: [128.0 ("Value") 0.0 ("Value") 0.0 ("Value")] -> w306
              tunnel: [64.0 ("Value") 0.5 ("Value") 1.0 ("Value")] -> w305
              frame "PWM" {
              }
              frame "Motor", Default {
              }
              frame "Analog Out" {
              }
            }
            n165 = property on="Motor" class="Clust (strict)"("Visible"=TRUE) -> ()  [unwired: 2 in, 2 out]
            n166 = property on="Value" class="Slide (strict)"("Value"=w306, "Scale.Minimum"=w308, "Scale.Maximum"=w307, "Scale.Increment"=w305) -> ()  [unwired: 2 in, 2 out]
            n167 = property on="On/Off" class="Bool (strict)"("Visible"=w310) -> ()  [unwired: 2 in, 2 out]
            n168 = property on="Test Slider" class="Slide (strict)"("Visible"=w310) -> ()  [unwired: 2 in, 2 out]
            n169 = property on="Test Ring" class="Ring (strict)"("Visible"=w310) -> ()  [unwired: 2 in, 2 out]
            n170 = property on="Rev/Fwd" class="Clust (strict)"("Visible"=w310) -> ()  [unwired: 2 in, 2 out]
          }
          frame "Servo" {
            w326 = FALSE ("Visible")
            n171 = call <vilib>:"NT Read Number.vi"("Name"=w328) -> ("Numeric"=w327:dbl)  [unwired: 9 in, 1 out]
            n172 = property on="Test Slider" class="Slide (strict)"("Visible"=TRUE, "Scale.Maximum"=170.0 ("Scale.Range:Maximum")) -> ()  [unwired: 2 in, 2 out]
            n173 = local write "Test Slider"(w327) -> ()
            n174 = property on="Motor" class="Clust (strict)"("Visible"=w326) -> ()  [unwired: 2 in, 2 out]
            n175 = property on="Rev/Fwd" class="Clust (strict)"("Visible"=w326) -> ()  [unwired: 2 in, 2 out]
            n176 = property on="On/Off" class="Bool (strict)"("Visible"=w326) -> ()  [unwired: 2 in, 2 out]
            n177 = property on="Test Ring" class="Ring (strict)"("Visible"=w326) -> ()  [unwired: 2 in, 2 out]
          }
          frame "Relay", "Solenoid" {
            w329 = FALSE ("Visible")
            n178 = property on="Motor" class="Clust (strict)"("Visible"=w329) -> ()  [unwired: 2 in, 2 out]
            n179 = property on="Test Slider" class="Slide (strict)"("Visible"=w329) -> ()  [unwired: 2 in, 2 out]
            n180 = Search and Replace String(input string=w330, search string="/Value  **", replace string="/Direction") -> (result string=w336:string)  [unwired: 5 in, 3 out]
            n181 = property on="Test Ring" class="Ring (strict)"("Visible"=w329) -> ()  [unwired: 2 in, 2 out]
            n182 = call <vilib>:"NT Read String.vi"("Name"=w336) -> ("String"=w334:string)  [unwired: 9 in, 1 out]
            n183 = Equal?(x="Both directions", y=w334) -> (x = y?=w332:bool)
            n184 = Not(x=w332) -> (.not. x?=w333:bool)
            n185 = property on="Rev/Fwd" class="Clust (strict)"("Visible"=w332) -> ()  [unwired: 2 in, 2 out]
            n186 = property on="On/Off" class="Bool (strict)"("Visible"=w333, "Caption.Text"=w331) -> ()  [unwired: 2 in, 2 out]
          }
          frame "Compressor", "Digital Out" {
            w339 = FALSE ("Visible")
            # "Get direction and finish"
            n187 = property on="Motor" class="Clust (strict)"("Visible"=w339) -> ()  [unwired: 2 in, 2 out]
            n188 = property on="Test Slider" class="Slide (strict)"("Visible"=w339) -> ()  [unwired: 2 in, 2 out]
            n189 = property on="Test Ring" class="Ring (strict)"("Visible"=w339) -> ()  [unwired: 2 in, 2 out]
            n190 = property on="On/Off" class="Bool (strict)"("Visible"=TRUE, "Caption.Text"=w340) -> ()  [unwired: 2 in, 2 out]
            n191 = property on="Rev/Fwd" class="Clust (strict)"("Visible"=FALSE) -> ()  [unwired: 2 in, 2 out]
          }
          frame "Camera" {
            n192 = call <vilib>:"Get Last Path Segment.vi"("String in"=w347) -> ("String out"=w348:string)  [unwired: 10 in]
            n193 = property on="On/Off" class="Bool (strict)"("Visible"=FALSE) -> ()  [unwired: 2 in, 2 out]
            n194 = property on="Motor" class="Clust (strict)"("Visible"=FALSE) -> ()  [unwired: 2 in, 2 out]
            n195 = property on="Rev/Fwd" class="Clust (strict)"("Visible"=FALSE) -> ()  [unwired: 2 in, 2 out]
            n196 = case shown="\"White Balance  **\"" w348 {
              tunnel: w347 -> [w354 w363 w372 w381 w390 _ w396]
              tunnel: w346 -> [w352 w360 w369 w378 w387 _ _]
              frame "Size  **" {
                n197 = Index Array(array=w352) -> (element=w351:cluster{string[]})  [unwired: 1 in]
                n198 = call <vilib>:"NT Read String.vi"("Name"=w354) -> ("String"=w353:string)  [unwired: 9 in, 1 out]
                n199 = Unbundle(w351) -> (w349:string[])
                n200 = Match First String(2:w349, 3:w353) -> (0:w350:i32)  [unwired: 1 out]
                n201 = property on="Test Ring" class="Ring (strict)"("Value"=w350, "Strings []"=w349) -> ()  [unwired: 2 in, 2 out]
                n202 = property on="Test Ring" class="Ring (strict)"("Visible"=TRUE) -> ()  [unwired: 2 in, 2 out]
                n203 = property on="Test Slider" class="Slide (strict)"("Visible"=FALSE) -> ()  [unwired: 2 in, 2 out]
              }
              frame "White Balance  **" {
                n204 = Index Array(array=w360, index=1) -> (element=w361:cluster{string[]})
                n205 = call <vilib>:"NT Read String.vi"("Name"=w363) -> ("String"=w362:string)  [unwired: 9 in, 1 out]
                n206 = Unbundle(w361) -> (w358:string[])
                n207 = Match First String(2:w358, 3:w362) -> (0:w357:i32)  [unwired: 1 out]
                n208 = property on="Test Ring" class="Ring (strict)"("Value"=w357, "Strings []"=w358) -> ()  [unwired: 2 in, 2 out]
                n209 = property on="Test Ring" class="Ring (strict)"("Visible"=TRUE) -> ()  [unwired: 2 in, 2 out]
                n210 = property on="Test Slider" class="Slide (strict)"("Visible"=FALSE) -> ()  [unwired: 2 in, 2 out]
              }
              frame "Exposure  **" {
                n211 = Index Array(array=w369, index=2) -> (element=w370:cluster{string[]})
                n212 = call <vilib>:"NT Read String.vi"("Name"=w372) -> ("String"=w371:string)  [unwired: 9 in, 1 out]
                n213 = Unbundle(w370) -> (w366:string[])
                n214 = Match First String(2:w366, 3:w371) -> (0:w367:i32)  [unwired: 1 out]
                n215 = property on="Test Ring" class="Ring (strict)"("Value"=w367, "Strings []"=w366) -> ()  [unwired: 2 in, 2 out]
                n216 = property on="Test Ring" class="Ring (strict)"("Visible"=TRUE) -> ()  [unwired: 2 in, 2 out]
                n217 = property on="Test Slider" class="Slide (strict)"("Visible"=FALSE) -> ()  [unwired: 2 in, 2 out]
              }
              frame "Exposure Priority  **" {
                n218 = Index Array(array=w378, index=3) -> (element=w379:cluster{string[]})
                n219 = call <vilib>:"NT Read String.vi"("Name"=w381) -> ("String"=w380:string)  [unwired: 9 in, 1 out]
                n220 = Unbundle(w379) -> (w375:string[])
                n221 = Match First String(2:w375, 3:w380) -> (0:w376:i32)  [unwired: 1 out]
                n222 = property on="Test Ring" class="Ring (strict)"("Value"=w376, "Strings []"=w375) -> ()  [unwired: 2 in, 2 out]
                n223 = property on="Test Ring" class="Ring (strict)"("Visible"=TRUE) -> ()  [unwired: 2 in, 2 out]
                n224 = property on="Test Slider" class="Slide (strict)"("Visible"=FALSE) -> ()  [unwired: 2 in, 2 out]
              }
              frame "Color Enable  **" {
                n225 = Index Array(array=w387, index=4) -> (element=w388:cluster{string[]})
                n226 = call <vilib>:"NT Read String.vi"("Name"=w390) -> ("String"=w389:string)  [unwired: 9 in, 1 out]
                n227 = Unbundle(w388) -> (w384:string[])
                n228 = Match First String(2:w384, 3:w389) -> (0:w385:i32)  [unwired: 1 out]
                n229 = property on="Test Ring" class="Ring (strict)"("Value"=w385, "Strings []"=w384) -> ()  [unwired: 2 in, 2 out]
                n230 = property on="Test Ring" class="Ring (strict)"("Visible"=TRUE) -> ()  [unwired: 2 in, 2 out]
                n231 = property on="Test Slider" class="Slide (strict)"("Visible"=FALSE) -> ()  [unwired: 2 in, 2 out]
              }
              frame Default {
                n232 = property on="Test Ring" class="Ring (strict)"("Visible"=FALSE) -> ()  [unwired: 2 in, 2 out]
                n233 = property on="Test Slider" class="Slide (strict)"("Visible"=FALSE) -> ()  [unwired: 2 in, 2 out]
              }
              frame "Brightness  **", "Color Level  **", "Compression  **", "FPS  **", "Sharpness  **" {
                n234 = call <vilib>:"NT Read Number.vi"("Name"=w396) -> ("Numeric"=w395:dbl)  [unwired: 9 in, 1 out]
                n235 = local write "Test Slider"(w395) -> ()
                n236 = property on="Test Slider" class="Slide (strict)"("Visible"=TRUE, "Scale.Maximum"=100.0 ("Scale.Range:Maximum")) -> ()  [unwired: 2 in, 2 out]
                n237 = property on="Test Ring" class="Ring (strict)"("Visible"=FALSE) -> ()  [unwired: 2 in, 2 out]
              }
            }
          }
        }
        n238 = property on="Progress" class="Clust (strict)"("Visible"=FALSE) -> ()  [unwired: 2 in, 2 out]
      }
      event "Test Name": Mouse Enter {
        # "Populate the ring with the list of tests"
        n239 = event-data() -> ()  [unwired: 1 in, 1 out]
        n240 = call <vilib>:"NT Read String Array.vi"("Name"="TestMode/TestList") -> ("String Array"=w404:string[])  [unwired: 9 in, 1 out]
        n241 = Build Array (concatenate)("Select the test to run...", w404) -> (w403:string[])
        n242 = property on="Test Name" class="Ring (strict)"("Strings []"=w403) -> ()  [unwired: 2 in, 2 out]
      }
      event "Test Name": Value Change {
        w406 = FALSE ("Visible")
        # "Tell the robot the test name to run"
        n243 = event-data() -> ("NewVal"=w410:u16)  [unwired: 1 in]
        n244 = property on="Test Name" class="Ring (strict)"() -> ("Strings []"=w411:string[])  [unwired: 2 in, 2 out]
        n245 = local write "Progress"(T6 {"Test Progress"=0, "Test Progress Text"=""} ("Progress")) -> ()
        n246 = Index Array(array=w411, index=w410) -> (element=w409:string)
        n247 = call <vilib>:"NT Write String.vi"("String"=w409, "Name"="TestMode/TestName") -> ()  [unwired: 9 in, 1 out]
        n248 = property on="Progress" class="Clust (strict)"("Visible"=TRUE) -> ()  [unwired: 2 in, 2 out]
        n249 = property on="Motor" class="Clust (strict)"("Visible"=w406) -> ()  [unwired: 2 in, 2 out]
        n250 = property on="Test Slider" class="Slide (strict)"("Visible"=w406) -> ()  [unwired: 2 in, 2 out]
        n251 = property on="On/Off" class="Bool (strict)"("Visible"=w406) -> ()  [unwired: 2 in, 2 out]
        n252 = property on="Rev/Fwd" class="Clust (strict)"("Visible"=w406) -> ()  [unwired: 2 in, 2 out]
        n253 = property on="Test Ring" class="Ring (strict)"("Visible"=w406) -> ()  [unwired: 2 in, 2 out]
      }
      event "Select Auto": Mouse Enter {
        # "Populate the combo box with the list of autonomous options"
        n254 = event-data() -> ()  [unwired: 1 in, 1 out]
        n255 = call <vilib>:"NT Read String Array.vi"("Name"="Auto List") -> ("String Array"=w413:string[])  [unwired: 9 in, 1 out]
        n256 = property on="Select Auto" class="CmbBox"("Strings[]"=w413) -> ()  [unwired: 2 in, 2 out]
      }
      event "Select Auto": Value Change {
        # "User modified the Auto Selection. Write to NT variable so robot knows."
        n257 = event-data() -> ("NewVal"=w416:string)  [unwired: 1 in]
        n258 = call <vilib>:"NT Write String.vi"("String"=w416, "Name"="Auto Selector") -> ()  [unwired: 9 in, 1 out]
      }
      event "Command Selection": Value Change {
        # "Get the params and show in table"
        n259 = event-data() -> ("NewVal"=w422:i32)  [unwired: 1 in]
        n260 = property on="Command Selection" class="MCListbox (strict)"() -> ("ItemNames"=w420:string[][])  [unwired: 2 in, 2 out]
        n261 = call <vilib>:"WPI_DashboardUpdate Command Params.vi"("NewVal"=w422, "Commands"=w420, "Param Tbl"=w421) -> ()  [unwired: 8 in, 1 out]
      }
      event "Execute Command": Value Change {
        # "Started one, Unique ID holds\nresponse"
        n262 = event-data() -> ()  [unwired: 1 in, 1 out]
        n263 = property on="Command Selection" class="MCListbox (strict)"() -> ("ItemNames"=w433:string[][])  [unwired: 2 in, 2 out]
        n264 = Index Array(array=w433, index (row)="Command Selection", index (col)=0) -> (element=w431:string)
        n265 = call <vilib>:"Invoke Commands.vi"("Command Params"="Command Params", "Function Name"=w431) -> ("Params"=w427:u8, "Started"=w426:bool)  [unwired: 7 in, 1 out]
        n266 = Array Subset(array="Command Params", length (row)=w427) -> (w428:string[][])  [unwired: 3 in]
        n267 = Select(t="Executing" ("Cmd Status"), s=w426, f="" ("Cmd Status")) -> (s? t:f=→"Cmd Status":string)
      }
      event "Command Selection": Double Click {
        n268 = event-data() -> ("Row"=w441:i32)  [unwired: 1 in]
        n269 = property on="Command Selection" class="MCListbox (strict)"() -> ("ItemNames"=w444:string[][])  [unwired: 2 in, 2 out]
        n270 = local read "Command Params"() -> (w440:string[][])
        n271 = Index Array(array=w444, index (row)=w441, index (col)=0) -> (element=w442:string)
        n272 = call <vilib>:"Invoke Commands.vi"("Command Params"=w440, "Function Name"=w442) -> ("Params"=w439:u8, "Started"=w434:bool)  [unwired: 7 in, 1 out]
        n273 = Array Subset(array=w440, length (row)=w439) -> (w438:string[][])  [unwired: 3 in]
        n274 = Select(t="Executing" ("Cmd Status"), s=w434, f="" ("Cmd Status")) -> (s? t:f=w435:string)
        n275 = local write "Cmd Status"(w435) -> ()
      }
      event "CheckList": Double Click {
        # "Shift clears all"
        # "Update symbols on the listbox"
        n276 = event-data() -> ("PlatMods.Shift"=w446:bool, "Row"=w448:i32)  [unwired: 1 in]
        n277 = case shown="True" w446 {
          tunnel: w448 -> [w452 _]
          tunnel: 1 -> [w451 _]
          frame False {
            n278 = property on="CheckList" class="LstBox (strict)"() -> ("Item Symbols"=w450:i32[])  [unwired: 2 in, 2 out]
            n279 = Replace Array Subset(array=w450, new element=w451, index=w452) -> (w449:i32[])
            n280 = property on="CheckList" class="LstBox (strict)"("Item Symbols"=w449) -> ()  [unwired: 2 in, 2 out]
          }
          frame True {
            w453 = 0 ("Top Row")
            n281 = property on="CheckList" class="LstBox (strict)"() -> ("Number of Rows"=w455:u32)  [unwired: 2 in, 2 out]
            n282 = Initialize Array(0, w455) -> (w454:i32[])
            n283 = property on="CheckList" class="LstBox (strict)"("Top Row"=w453, "Value"=w453, "Item Symbols"=w454) -> ()  [unwired: 2 in, 2 out]
          }
        }
      }
      event "CheckList": Key Down {
        # "Update symbols on the listbox\nLeft and right keys check and uncheck"
        n284 = event-data() -> ("VKey"=w459:T23)  [unwired: 1 in]
        n285 = case shown="\"Left\", \"Right\"" w459 {
          selector: w459 -> [w464 _]
          tunnel: eventvkey."Left" ("VKey") -> [w462 _]
          frame "Left", "Right" {
            n286 = Equal?(x=w462, y=w464) -> (x = y?=w463:bool)
            n287 = Select(t=0, s=w463, f=1) -> (s? t:f=w465:i32)
            n288 = property on="CheckList" class="LstBox (strict)"() -> ("Item Symbols"=w468:i32[])  [unwired: 2 in, 2 out]
            n289 = Replace Array Subset(array=w468, new element=w465, index="CheckList") -> (w467:i32[])
            n290 = property on="CheckList" class="LstBox (strict)"("Item Symbols"=w467) -> ()  [unwired: 2 in, 2 out]
          }
          frame Default {
          }
        }
      }
      event "Motor.Enable": Value Change {
        # "When the test mode otor enable helper is set, update that\ntree row item's value"
        n291 = event-data() -> ("NewVal"=w474:bool)  [unwired: 1 in]
        n292 = Unbundle("Motor") -> ("Value"=w473:dbl)  [unwired: 1 out]
        n293 = Select(t=w473, s=w474, f=0.0) -> (s? t:f=w471:dbl)
        n294 = call <vilib>:"NT Write Number.vi"("Numeric"=w471, "Name"=w470) -> ()  [unwired: 9 in, 1 out]
      }
      event "Test Slider": Value Change {
        # "When the test mode slider helper is set, update that\ntree row item's value"
        n295 = event-data() -> ("NewVal"=w477:dbl)  [unwired: 1 in]
        n296 = call <vilib>:"NT Write Number.vi"("Numeric"=w477, "Name"=w478) -> ()  [unwired: 9 in, 1 out]
      }
      event "On/Off": Value Change {
        # "When the test mode on/off helper value is set, update that\ntree row item's value"
        n297 = event-data() -> ("NewVal"=w482:bool)  [unwired: 1 in]
        n298 = Boolean To (0,1)(Boolean=w482) -> (0, 1=w481:i16)
        n299 = call <vilib>:"NT Write Number.vi"("Numeric"=w481, "Name"=w480) -> ()  [unwired: 9 in, 1 out]
      }
      event "Rev/Fwd": Value Change {
        # "When the test mode helper value for relays is set, update that\ntree row item's value"
        n300 = event-data() -> ("NewVal.Forward"=w490:bool, "NewVal.Reverse"=w489:bool)  [unwired: 1 in]
        n301 = Boolean To (0,1)(Boolean=w490) -> (0, 1=w486:i16)
        n302 = Boolean To (0,1)(Boolean=w489) -> (0, 1=w488:i16)
        n303 = Negate(x=w488) -> (-x=w487:i16)
        n304 = Add(x=w486, y=w487) -> (x+y=w485:i16)
        n305 = call <vilib>:"NT Write Number.vi"("Numeric"=w485, "Name"=w484) -> ()  [unwired: 9 in, 1 out]
      }
      event "Test Ring": Value Change {
        # "When a test mode helper value is selected from the ring,\nset the tree item's variable to the string value"
        n306 = event-data() -> ("NewVal"=w494:u16)  [unwired: 1 in]
        n307 = property on="Test Ring" class="Ring (strict)"() -> ("Strings []"=w495:string[])  [unwired: 2 in, 2 out]
        n308 = Index Array(array=w495, index=w494) -> (element=w493:string)
        n309 = call <vilib>:"NT Write String.vi"("String"=w493, "Name"=w492) -> ()  [unwired: 9 in, 1 out]
      }
      event "Rec Mode": Value Change {
        # "Update globals for recording mode and path to read log from.\nClear when logging and let NetworkTables set path for vision to\nuse."
        n310 = event-data() -> ("NewVal"=w506:enum32{"Stop", "Record", "Playback"})  [unwired: 1 in]
        n311 = global write "WPI_DashboardLogging Global.vi" "Logging Filename"(path "") -> ()
        n312 = global write "WPI_DashboardLogging Global.vi" "Recording"(w506) -> ()
        n313 = case shown="\"Playback\"" w506 {
          tunnel: w505 -> [_ w508 w517]
          tunnel: [_ _ w516] -> w503
          tunnel: [_ _ w515] -> _
          tunnel: w501 -> [_ _ w513]
          tunnel: cluster{i32, i32} {-250, 170} -> [_ _ w512]
          tunnel: [_ _ T24 {"Image Size"=TRUE, "Image Type"=TRUE, "Pixel Value"=TRUE, "ROI Information"=TRUE, "Zoom Factor"=FALSE} ("Image Information Shown:All Elements")] -> w496
          tunnel: [_ _ TRUE ("Zoom Factor")] -> w497
          tunnel: w499 -> [_ _ w509]
          frame Default {
          }
          frame "Stop", "Record" {
            # "Place Window too"
            n314 = invoke class="VI" method="FP.Close"(reference=w508) -> (reference out=w507:refnum<vi>)  [unwired: 2 in, 2 out]
            n315 = invoke class="VI" method="Abort VI"(reference=w507) -> ()  [unwired: 2 in, 3 out]
          }
          frame "Playback" {
            n316 = call "Open Playback Panel.vi"("Offset"=w512, "DB VI Ref"=w513, "Playback in"=w517) -> ("Playback out"=w514:refnum<vi>)  [unwired: 8 in]
            n317 = register-events(w514, w509) -> (reference out=w516:refnum<event-registration>, error out=w515:errorcluster)  [unwired: 2 in]
          }
        }
        n318 = property on="Camera Image Right" class="ImageControl"("Image Information Shown"=w496, "Image Information Visible"=w497) -> ()  [unwired: 2 in, 2 out]
        n319 = property on="Camera Image" class="ImageControl"("Image Information Shown"=w496, "Image Information Visible"=w497) -> ()  [unwired: 2 in, 2 out]
        n320 = call <vilib>:"WPI_DashboardNT Log FieldName Cache.vi"("Operation"=enum16{"Lookup/Add", "Index", "Clear"}."Clear") -> ()  [unwired: 8 in, 3 out]
      }
      event Panel Close {
        w519 = enum32{"Stop", "Record", "Playback"}."Stop" ("Rec Mode")
        # "Playback window has been closed, abort"
        n321 = event-data() -> ()  [unwired: 1 in, 4 out]
        n322 = local write "Rec Mode"(w519) -> ()
        n323 = global write "WPI_DashboardLogging Global.vi" "Recording"(w519) -> ()
      }
      event Panel Close {
        # "Abort playback window and ourself"
        n324 = event-data() -> ()  [unwired: 1 in, 4 out]
        n325 = invoke class="VI" method="FP.Close"(reference=w523) -> (reference out=w522:refnum<vi>)  [unwired: 2 in, 2 out]
        n326 = invoke class="VI" method="Abort VI"(reference=w522) -> (error out=w521:errorcluster)  [unwired: 2 in, 2 out]
        n327 = invoke class="VI" method="Abort VI"(error in=w521) -> ()  [unwired: 2 in, 3 out]
      }
      event User Event {
        n328 = event-data() -> ("IDs"=w530:cluster{"RPC field ID":u16, "Unique ID":u16}, "String"=w529:string)  [unwired: 1 in]
        n329 = Bundle("IDs"=w530, "String"=w529) -> (w528:T9)  [unwired: 1 in]
        n330 = call <vilib>:"Retrieve RPC Response.vi"("RPC Response"=w528) -> ("Output"=w526:string[][])  [unwired: 10 in]
        n331 = Build Array (concatenate)(w524, w526) -> (w525:string[][])
        n332 = local write "Command Params"(w525) -> ()
        n333 = local write "Cmd Status"("" ("Cmd Status")) -> ()
      }
      event "Tree": Double Click {
        n334 = event-data() -> ("PlatMods"=w536:T27, "Tag"=w533:string)  [unwired: 1 in]
        n335 = Unbundle(w536) -> ("Shift"=w535:bool)  [unwired: 4 out]
        n336 = String Subset(string=w533, length (rest)=1 ("length (rest)")) -> (substring=w532:string)  [unwired: 1 in]
        n337 = Not(x=w535) -> (.not. x?=w534:bool)
        n338 = case shown="\"/\"" w532 {
          tunnel: w533 -> [_ w539]
          tunnel: w534 -> [_ w538]
          frame Default {
          }
          frame "/" {
            n339 = call <vilib>:"NT Update Persistence.vi"("Persistence"=w538, "Name"=w539) -> ()  [unwired: 9 in, 1 out]
          }
        }
      }
    }
  }
  n340 = while {
    tunnel: w65 -> [w541]
    i -> [w544]
    stop <- FALSE stop-if-true
    n341 = Wait (ms)(milliseconds to wait=u32 100) -> ()  [unwired: 1 out]
    n342 = case shown="\"Playback\"" "Rec Mode" {
      tunnel: w544 -> [_ _ w559]
      tunnel: [u32 2829099 ("Base Color") u32 11141120 ("Target Color") w548] -> w540
      frame "Stop", Default {
        # "Reset the color, extra updates don't cost much"
      }
      frame "Record" {
      }
      frame "Playback" {
        # "Playback"
        n343 = Quotient & Remainder(x=w559, y=u32 50 ("milliseconds to wait")) -> (x-y*floor(x/y)=w555:u32)  [unwired: 1 out]
        n344 = Divide(x=w555, y=u32 50 ("milliseconds to wait")) -> (x/y=w552:dbl)
        n345 = Multiply(x=6.283185307179586, y=w552) -> (x*y=w557:dbl)
        n346 = Sine(x=w557) -> (sin(x)=w556:dbl)
        n347 = Absolute Value(x=w556) -> (abs(x)=w549:dbl)
        n348 = call "Interpolate RGB Color.vi"("Proportion"=w549, "Target Color"=u32 30976, "Base Color"=u32 2829099) -> ("Result Color"=w548:u32)  [unwired: 8 in]
      }
    }
    n349 = property class="Pane"(reference=w541, "PaneColor"=w540) -> ()  [unwired: 1 in, 2 out]
  }
  n350 = local write "Dashboard Tab"(T2."Drive" ("Dashboard Tab")) -> ()
  n351 = property on="On/Off" class="Bool (strict)"("Visible"=w36) -> ()  [unwired: 2 in, 2 out]
  n352 = property on="Motor" class="Clust (strict)"("Visible"=w36) -> ()  [unwired: 2 in, 2 out]
  n353 = property on="Progress" class="Clust (strict)"("Visible"=w36) -> ()  [unwired: 2 in, 2 out]
  n354 = property on="Test Ring" class="Ring (strict)"("Visible"=w36) -> ()  [unwired: 2 in, 2 out]
  n355 = property on="Rev/Fwd" class="Clust (strict)"("Visible"=w36) -> ()  [unwired: 2 in, 2 out]
  n356 = while {
    tunnel: u16 1741 ("timeout ms (25000)") -> [w561]
    stop <- FALSE stop-if-true
    n357 = TCP Create Listener(10:w561) -> (0:w560:errorcluster, 3:w562:refnum<k5>)  [unwired: 4 in, 1 out]
    n358 = case shown="No Error" w560 {
      selector: w560 -> [w564 _]
      tunnel: w562 -> [w565 _]
      frame No Error {
        n359 = while {
          tunnel: w565 -> [w568]
          tunnel: w564 -> [w567]
          stop <- FALSE stop-if-true
          n360 = TCP Wait On Listener(8:w567, 11:w568) -> (0:w569:errorcluster, 4:w570:refnum<k5>)  [unwired: 2 in, 3 out]
          n361 = local write "TCP"(w570) -> ()
          n362 = case shown="No Error" w569 {
            frame No Error {
            }
            frame Error {
              n363 = Wait (ms)(milliseconds to wait=u32 1000) -> ()  [unwired: 1 out]
            }
          }
        }
      }
      frame Error {
        n364 = Wait (ms)(milliseconds to wait=u32 1000) -> ()  [unwired: 1 out]
      }
    }
  }
  n365 = local write "Command Selection"(u16 0 ("milliseconds to wait")) -> ()
  n366 = local write "Command Params"(string[][] [] ("Command Params")) -> ()
  n367 = global write "WPI_DashboardLogging Global.vi" "Recording"(w59) -> ()
  n368 = local write "Rec Mode"(w59) -> ()
  n369 = call <vilib>:"NT Write String.vi"("String"="Select Auto", "Name"="Auto Selector") -> ()  [unwired: 9 in, 1 out]
